vi "AddRecord.vi"(0 "reference in":refnum<class "CustomersData.lvclass">, 1 "Customer":string, 5 "error in (no error)":errorcluster) -> (14 "reference out":refnum<class "CustomersData.lvclass">, 19 "error out":errorcluster)   [LabVIEW 2020, in "CustomersData.lvclass"]
uses:
  CustomersData.lvclass
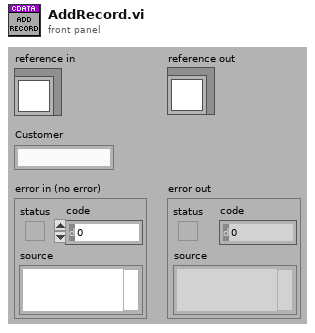
[diagram p1: front panel]
types:
  T1 = typedef "CustomersData.lvclass/ObjectAttributes.ctl" = cluster{"_customers":string[], "_current":i32}
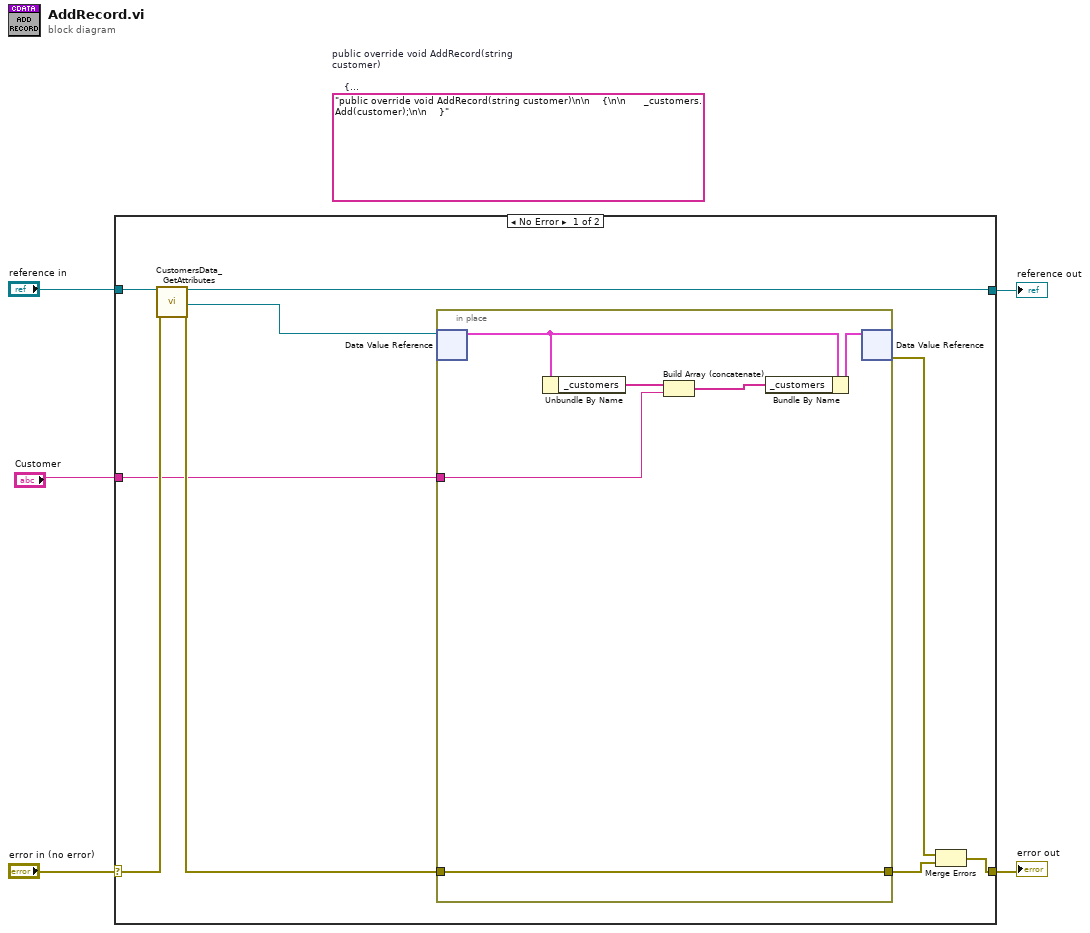
[diagram p0: block diagram]
diagram:
  (unwired) "public override void AddRecord(string customer)\n\n    {\n\n      _customers.Add(customer);\n\n    }"  # public override void AddRecord(string customer)      {        _customers.Add(customer);      }
  n1 = case shown="No Error" "error in (no error)" {
    selector: "error in (no error)" -> [w13 w22]
    tunnel: [w11 w22] -> w4
    tunnel: [w10 w21] -> w2
    tunnel: "reference in" -> [w14 w21]
    tunnel: "Customer" -> [w6 _]
    frame No Error {
      n2 = call "CustomersData_GetAttributes.vi"("reference in"=w14, "error in (no error)"=w13) -> ("reference out"=w10:refnum<class "CustomersData.lvclass">, "DataRef"=w9:refnum<data-value>, "error out"=w8:errorcluster)  [unwired: 14 in, 1 out]
      n3 = in-place {
        in-place-border: w8 -> [w19]
        in-place-border: [w19] -> w7
        in-place-border: w6 -> [w15]
        n4 = in-place-dvr #1(w9) -> (w18:T1)  [unwired: 1 out]
        n5 = Unbundle By Name(w18) -> ("_customers"=w17:string[])
        n6 = Build Array (concatenate)(w17, w15) -> (w16:string[])
        n7 = Bundle By Name(cluster=w18, "_customers"=w16) -> (w20:T1)
        n8 = in-place-dvr #1(w20) -> (w12:errorcluster)  [unwired: 1 out]
      }
      n9 = Merge Errors(w12, w7) -> (w11:errorcluster)
    }
    frame Error {
    }
  }
  "error out" <- w4
  "reference out" <- w2
